vi "Library_Status_init.vi"(8 "error in (no error)":errorcluster) -> (0 "error out":errorcluster)   [LabVIEW 2013]
uses:
  My Computer/Controls/Sepios_status.ctl
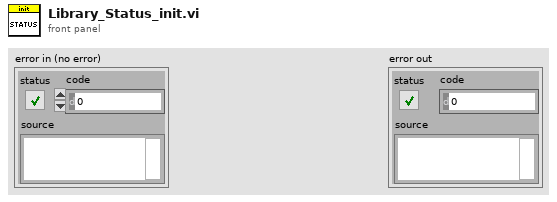
[diagram p1: front panel]
types:
  T1 = typedef "Sepios_status.ctl" = enum16{"Standby", "Running", "Filming", "Error"}
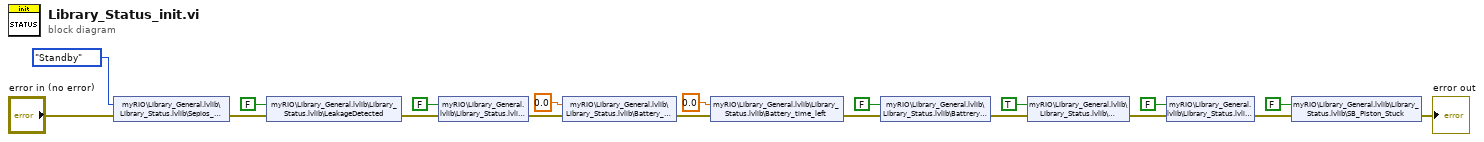
[diagram p0: block diagram]
diagram:
  n1 = shared-variable "myRIO\\Library_General.lvlib\\Library_Status.lvlib\\Sepios_Status"(Sepios_status."Standby" ("Sepios_Status"), error in="error in (no error)") -> (error out=w15:errorcluster)
  n2 = shared-variable "myRIO\\Library_General.lvlib\\Library_Status.lvlib\\LeakageDetected"(FALSE ("LeakageDetected"), error in=w15) -> (error out=w17:errorcluster)
  n3 = shared-variable "myRIO\\Library_General.lvlib\\Library_Status.lvlib\\tooDeep"(FALSE ("tooDeep"), error in=w17) -> (error out=w13:errorcluster)
  n4 = shared-variable "myRIO\\Library_General.lvlib\\Library_Status.lvlib\\Battery_Level"(0.0 ("Battery_Level"), error in=w13) -> (error out=w12:errorcluster)
  n5 = shared-variable "myRIO\\Library_General.lvlib\\Library_Status.lvlib\\Battery_time_left"(0.0 ("Battery_time_left"), error in=w12) -> (error out=w11:errorcluster)
  n6 = shared-variable "myRIO\\Library_General.lvlib\\Library_Status.lvlib\\Battrery_Full"(FALSE ("Battrery_Full"), error in=w11) -> (error out=w3:errorcluster)
  n7 = shared-variable "myRIO\\Library_General.lvlib\\Library_Status.lvlib\\CameraOn"(TRUE ("CameraOn"), error in=w3) -> (error out=w2:errorcluster)
  n8 = shared-variable "myRIO\\Library_General.lvlib\\Library_Status.lvlib\\LaserOn"(FALSE ("LaserOn"), error in=w2) -> (error out=w1:errorcluster)
  n9 = shared-variable "myRIO\\Library_General.lvlib\\Library_Status.lvlib\\SB_Piston_Stuck"(FALSE ("SB_Piston_Stuck"), error in=w1) -> (error out=→"error out":errorcluster)
